vi "ReadRGB.vi"() -> ()   [LabVIEW 2012]
uses:
  <vilib>/picture/picture.llb/Draw True-Color Pixmap.vi
panel:
  out "Height":u32[][](graph)
  out "Offset4":i64
  in  "Gap3":i64=796
  out "Intensity":u16[][](graph)
  in  "Gap2":i64=796
  in  "Gap1":i64=20
  out "Offset3":i64
  out "Offset2":i64
  out "RGB2":picture
  out "RGB1":picture
  in  "SizeY":i64=768
  in  "SizeX":i64=1024
  in  "Offset":i64=752
  in  "Path1":path
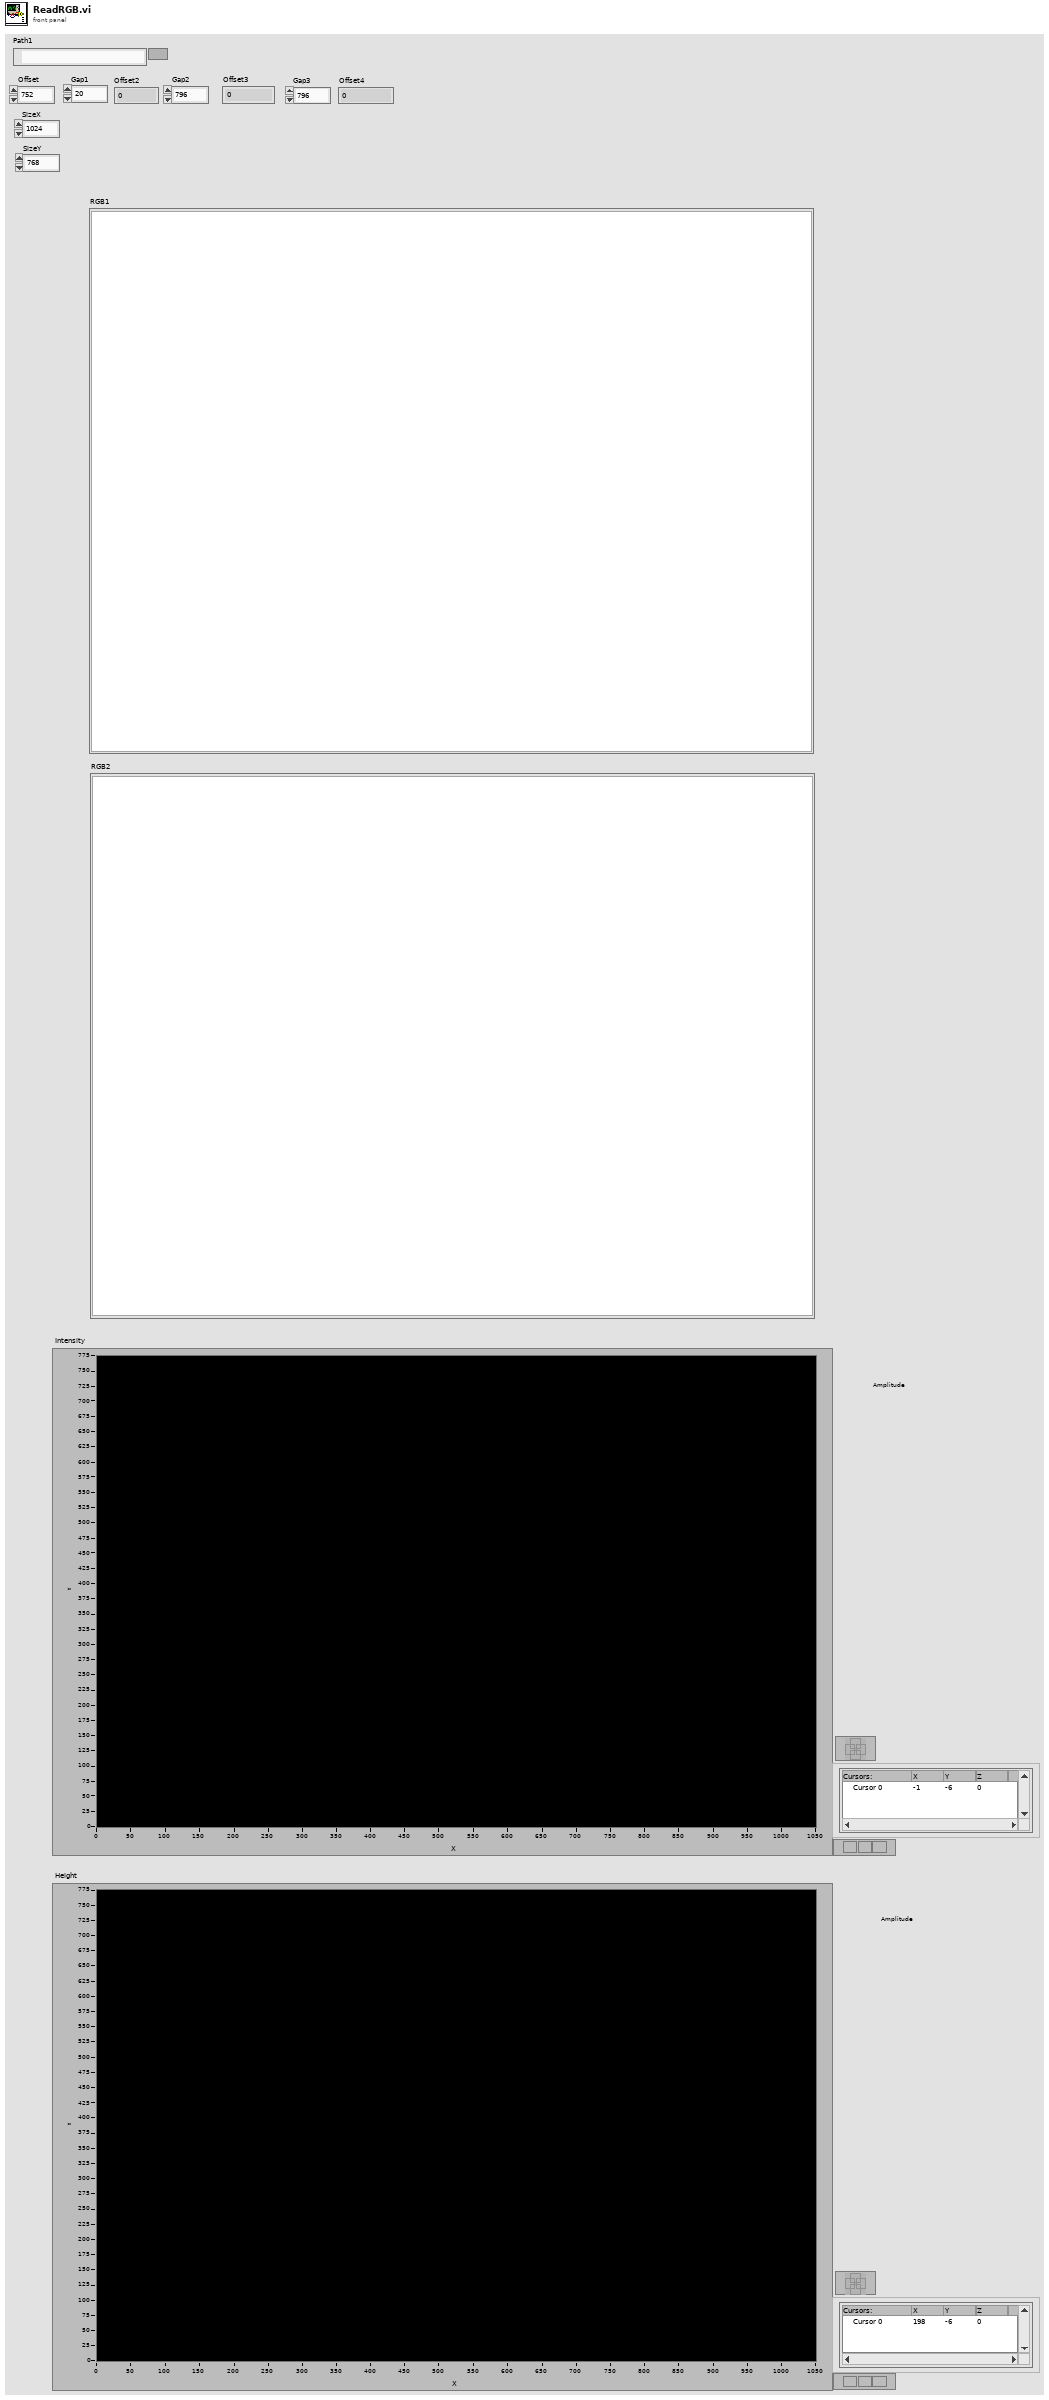
[diagram p1: front panel]
types:
  T1 = enum16{"big-endian, network order", "native, host order", "little-endian"}
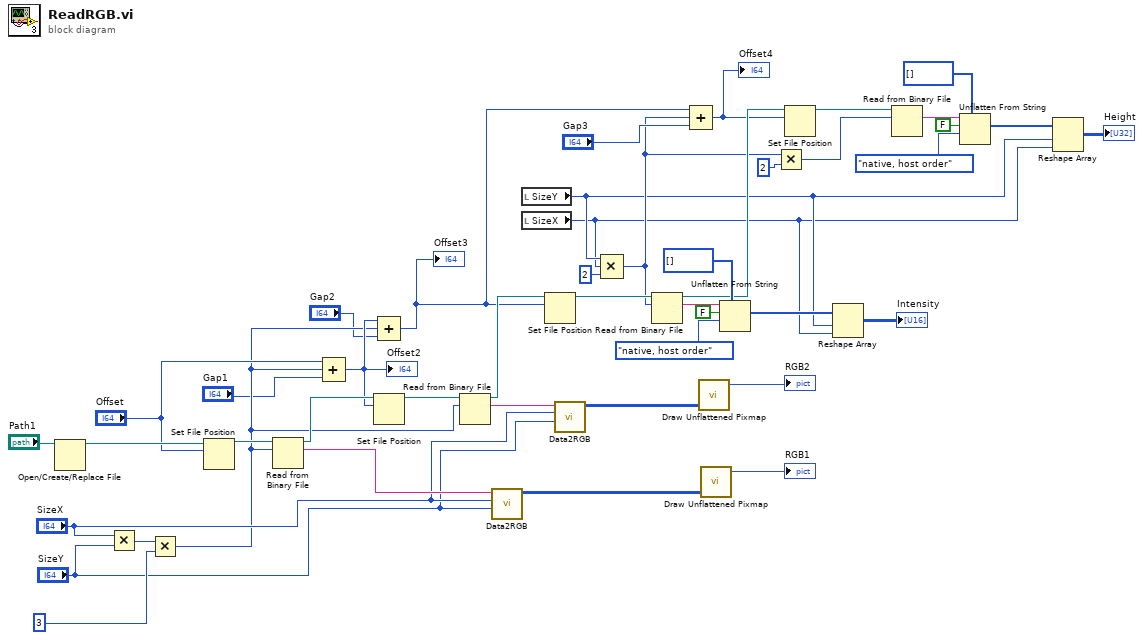
[diagram p0: block diagram]
diagram:
  n1 = Open/Create/Replace File(file path (use dialog)="Path1") -> (refnum out=w43:refnum<file>)  [unwired: 5 in, 2 out]
  n2 = Multiply(x="SizeX", y="SizeY") -> (x*y=w42:i64)
  n3 = Multiply(x=w42, y=i64 3) -> (x*y=w28:i64)
  n4 = Set File Position(offset (in bytes) (0)="Offset", refnum=w43) -> (refnum out=w44:refnum<file>)  [unwired: 2 in, 1 out]
  n5 = Read from Binary File(10:w28, 11:w44) -> (2:w41:string, 3:w37:refnum<file>)  [unwired: 4 in, 2 out]
  n6 = Compound Arithmetic op=ADD("Offset", w28, "Gap1") -> (w29:i64)
  "Offset2" <- w29
  n7 = Set File Position(offset (in bytes) (0)=w29, refnum=w37) -> (refnum out=w36:refnum<file>)  [unwired: 2 in, 1 out]
  n8 = Compound Arithmetic op=ADD(w29, w28, "Gap2") -> (w16:i64)
  "Offset3" <- w16
  n9 = Read from Binary File(10:w28, 11:w36) -> (2:w35:string, 3:w26:refnum<file>)  [unwired: 4 in, 2 out]
  n10 = call "Data2RGB.vi"("SizeY"="SizeY", "SizeX"="SizeX", "Data"=w41) -> ("RGBarray"=w39:u32[][])  [unwired: 8 in]
  n11 = local read "SizeY"() -> (w3:i64)
  n12 = local read "SizeX"() -> (w2:i64)
  n13 = Set File Position(offset (in bytes) (0)=w16, refnum=w26) -> (refnum out=w27:refnum<file>)  [unwired: 2 in, 1 out]
  n14 = call "Data2RGB.vi"("SizeY"="SizeY", "SizeX"="SizeX", "Data"=w35) -> ("RGBarray"=w34:u32[][])  [unwired: 8 in]
  n15 = Compound Arithmetic op=MULTIPLY(w3, w2, i64 2 ("value")) -> (w7:i64)
  n16 = Read from Binary File(10:w7, 11:w27) -> (2:w23:string, 3:w9:refnum<file>)  [unwired: 4 in, 2 out]
  n17 = Compound Arithmetic op=ADD(w16, w7, "Gap3") -> (w8:i64)
  "Offset4" <- w8
  n18 = call-poly <vilib>:"Draw Unflattened Pixmap.vi"("data (RGB format)"=w34) -> ("new picture"=→"RGB2":picture)  [unwired: 8 in]
  n19 = call-poly <vilib>:"Draw Unflattened Pixmap.vi"("data (RGB format)"=w39) -> ("new picture"=→"RGB1":picture)  [unwired: 8 in]
  n20 = Unflatten From String(type=u16[] [], binary string=w23, data includes array or string size? (T)=FALSE, byte order (0:big-endian, network order)=T1."native, host order") -> (value=w21:u16[])  [unwired: 1 in, 2 out]
  n21 = Multiply(x=w7, y=i64 2) -> (x*y=w5:i64)
  n22 = Set File Position(offset (in bytes) (0)=w8, refnum=w9) -> (refnum out=w10:refnum<file>)  [unwired: 2 in, 1 out]
  n23 = Reshape Array(w21, w3, w2) -> (→"Intensity":u16[][])
  n24 = Read from Binary File(10:w5, 11:w10) -> (2:w11:string)  [unwired: 4 in, 3 out]
  n25 = Unflatten From String(type=u32[] [], binary string=w11, data includes array or string size? (T)=FALSE, byte order (0:big-endian, network order)=T1."native, host order") -> (value=w4:u32[])  [unwired: 1 in, 2 out]
  n26 = Reshape Array(w4, w3, w2) -> (→"Height":u32[][])
